vi "Read Message Header.vi"(11 "Message header":string) -> (3 "Message Size":u64)   [LabVIEW 2024, in "Ramses Framework.lvlib"]
doc: "Reads the message header and converts it into a U64 message size."
uses:
  Ramses Framework.lvlib
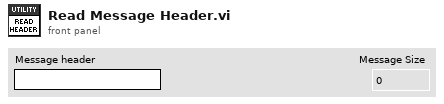
[diagram p1: front panel]
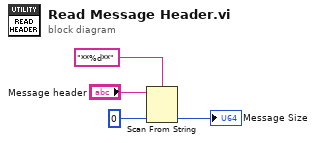
[diagram p0: block diagram]
diagram:
  n1 = Scan From String(format string="**%d**", input string="Message header", default 1=u64 0 ("unsigned 64bit integer")) -> (output 1=→"Message Size":u64)  [unwired: 2 in, 3 out]
